vi "Parse Data JSON.vi"(8 "error in (no error)":errorcluster, 10 "JSON String":string, 11 "Hello in":refnum<class "Hello.lvclass">) -> (0 "error out":errorcluster, 1 "Typed?":bool, 2 "Typed Message":refnum<class "Response.lvclass">, 3 "Hello out":refnum<class "Hello.lvclass">)   [LabVIEW 2020, in "obs-websocket.lvlib" / "Hello.lvclass"]
uses:
  Hello.lvclass
  Response/Response.lvclass
  Authentication.ctl
  Hello.lvclass/Hello.ctl
  72354c48-2640-47a5-b646-1a626b898f5a.vi
  <vilib>/JDP Science/JSONtext/JSON text to Variant.vi
  <vilib>/JDP Science/JSONtext/LVClass Serializer/JSONtext LVClass Serializer.lvclass
  obs-websocket.lvlib
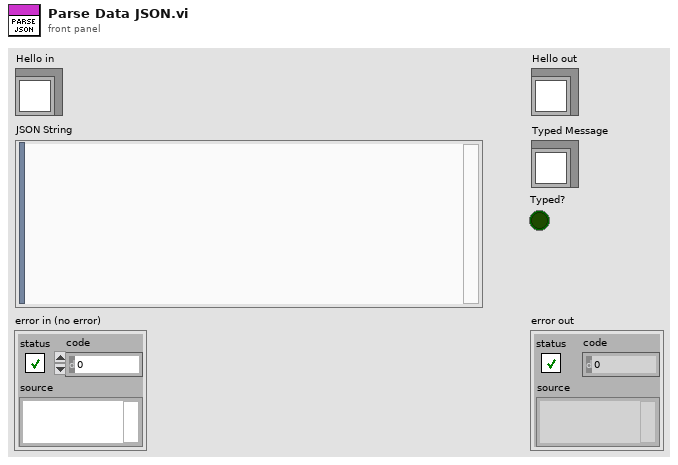
[diagram p1: front panel]
types:
  T1 = typedef "obs-websocket.lvlib/Authentication.ctl" = cluster{"Has Authentication":bool, "Salt":string, "Challenge":string}
  T2 = cluster{"obsWebSocketVersion":string, "rpcVersion":i32, "authentication":cluster{"salt":string, "challenge":string}}
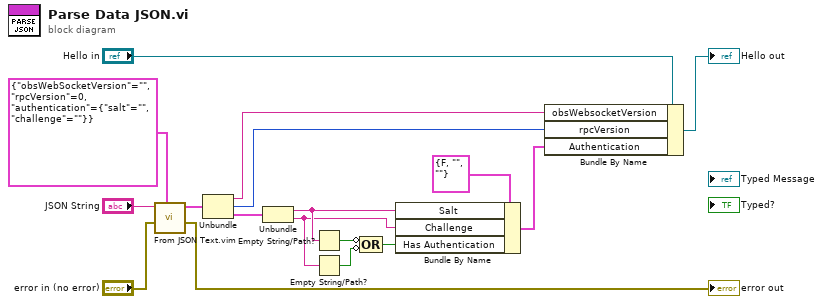
[diagram p0: block diagram]
diagram:
  n1 = call "From JSON Text.vim"("Data Type and Default Value"=T2 {"obsWebSocketVersion"="", "rpcVersion"=0, "authentication"={"salt"="", "challenge"=""}}, "error in (no error)"="error in (no error)", "JSON"="JSON String") -> ("error out"=→"error out":errorcluster, "Data out"=w12:T2)  [unwired: 7 in]
  n2 = Unbundle(w12) -> ("obsWebSocketVersion"=w7:string, "rpcVersion"=w6:i32, "authentication"=w11:cluster{"salt":string, "challenge":string})
  n3 = Unbundle(w11) -> ("salt"=w5:string, "challenge"=w4:string)
  n4 = Empty String/Path?(string/path=w5) -> (empty?=w10:bool)
  n5 = Empty String/Path?(string/path=w4) -> (empty?=w9:bool)
  n6 = Compound Arithmetic op=OR(invert w10, invert w9) -> (w3:bool)
  n7 = Bundle By Name(cluster=T1 {"Has Authentication"=FALSE, "Salt"="", "Challenge"=""} ("Authentication"), "Salt"=w5, "Challenge"=w4, "Has Authentication"=w3) -> (w15:T1)
  n8 = Bundle By Name(cluster="Hello in", "obsWebsocketVersion"=w7, "rpcVersion"=w6, "Authentication"=w15) -> (→"Hello out":refnum<class "Hello.lvclass">)
